vi "send channel config file.vi"(6 "messageHandler":T2 {"params"."controlChannels"."ballControl" items=["Module6/output0", "Module6/output1", "Module6/output2", "Module6/output3", "Not-Used"]; "params"."controlChannels"."butterflyControl" items=["Module6/output0", "Module6/output1", "Module6/output2", "Module6/output3", "Not-Used"]; "params"."controlChannels"."speedControl" items=["Module6/output0", "Module6/output1", "Module6/output2", "Module6/output3", "Not-Used"]}, 11 "Queues":T1) -> ()   [LabVIEW 2018]
uses:
  type defs/message handler data.ctl
  customVI/liveData/state.ctl
  type defs/Queues.ctl
types:
  T1 = typedef "Queues.ctl" = cluster{"messageHandler":refnum<queue>, "comms":refnum<queue>, "dataStream":refnum<queue>, "dataProcessor":refnum<queue>, "fileIO":refnum<queue>, "userInterface":refnum<queue>, "errors":refnum<queue>, "customCompressor":refnum<queue>}
  T2 = typedef "message handler data.ctl" = cluster{"params":cluster{"configFileID":u32, "configFilePath":path, "channelConfigFilePath":path, "incidentLogfile":path, "controlChannels":cluster{"ballControl":u16, "butterflyControl":u16, "speedControl":u16}, "pulsatorVIPath":path, "customVIPath":path, "HowdenAir":cluster{"vent Howden":bool, "Howden%":dbl}}, "vars":cluster{"commsStatus":bool[], "controlIndex":cluster{"ballControl":u16, "butterflyControl":u16, "speedControl":u16}, "customVIRef":refnum<vi>, "Interlocks":cluster{"gearboxOil":bool, "bearingOil":bool, "gearboxAir":bool}, "motorRunning":bool, "liveDataQ":refnum<queue>[]}}
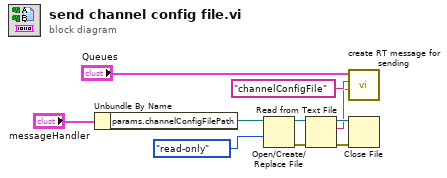
[diagram p0: block diagram]
diagram:
  n1 = Unbundle By Name("messageHandler") -> ("params.channelConfigFilePath"=w8:path)
  n2 = Open/Create/Replace File(file path (use dialog)=w8, access (0:read/write)=enum16{"read/write", "read-only", "write-only"}."read-only") -> (refnum out=w6:refnum<file>, error out=w7:errorcluster)  [unwired: 4 in, 1 out]
  n3 = Read from Text File(file (use dialog)=w6, error in=w7) -> (refnum out=w4:refnum<file>, text=w2:string, error out=w5:errorcluster)  [unwired: 2 in, 1 out]
  n4 = call "create RT message for sending.vi"("RT data"=w2, "RT message"="channelConfigFile", "Queues in"="Queues") -> ()  [unwired: 8 in, 1 out]
  n5 = Close File(refnum=w4, error in=w5) -> ()  [unwired: 2 out]
